vi "TemperatureProfileDesigner.vi"() -> (3 "ShcemeCluster":cluster{"Time":dbl, "Voltage":dbl}[](array[cluster]))   [LabVIEW 2023]
uses:
  <vilib>/Analysis/1siggen.llb/Ramp Pattern by Samples.vi
  <vilib>/Analysis/1siggen.llb/Ramp Pattern by Delta.vi
  <vilib>/Analysis/NI_AALBase.lvlib
panel:
  in  "Time (s)":dbl
  out "XY Graph":cluster{dbl[], dbl[]}(graph)
  in  "Schedule":bool
  in  "Ramp points (s)":i16 min=0 max=7200 step=1
  in  "Step / Ramp":bool
  in  "Up & Down":bool
  in  "Step":dbl min=0.0 max=450.0 step=1.0
  in  "Stop":dbl=20.0 min=20.0 max=450.0 step=1.0
  in  "Start":dbl=20.0 min=20.0 max=450.0 step=1.0
  # "Temperature Profile Designer"
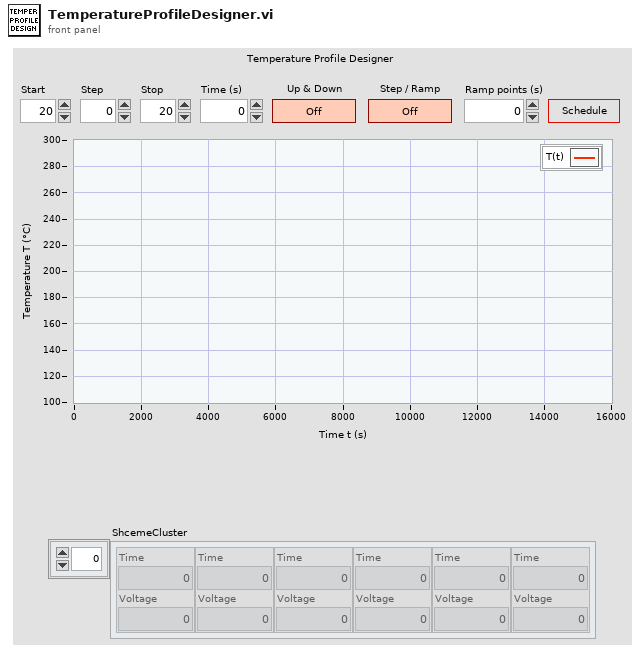
[diagram p1: front panel]
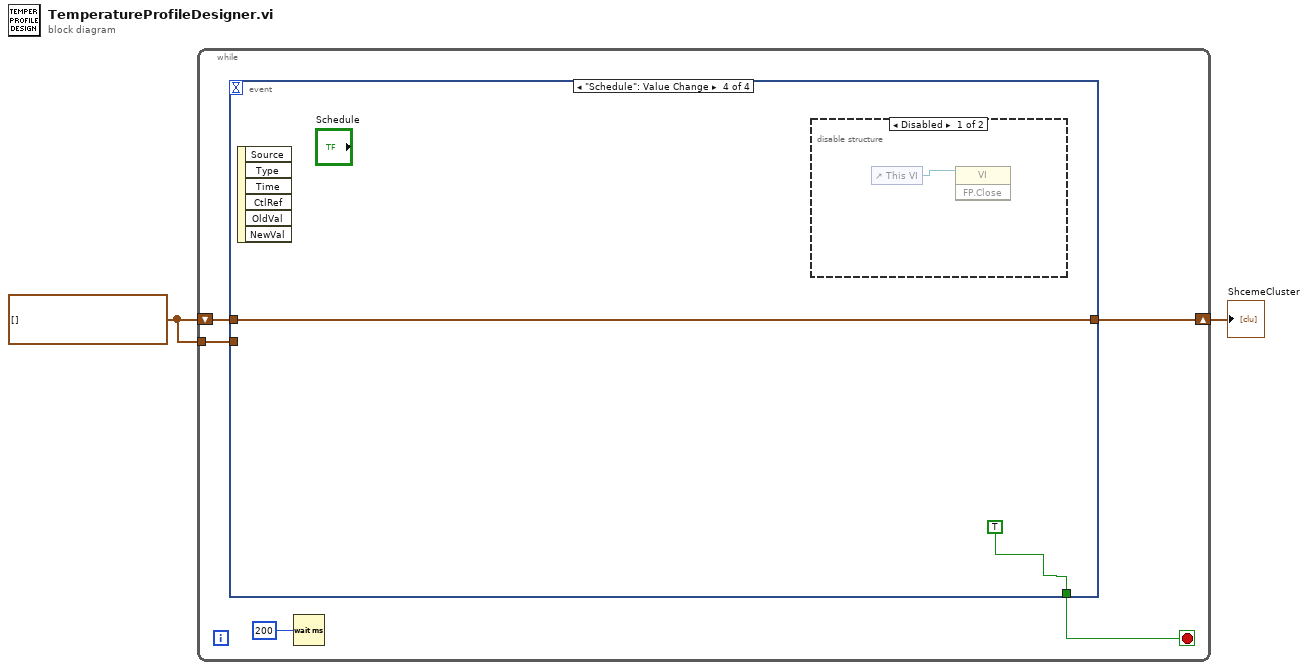
[diagram p0: block diagram]
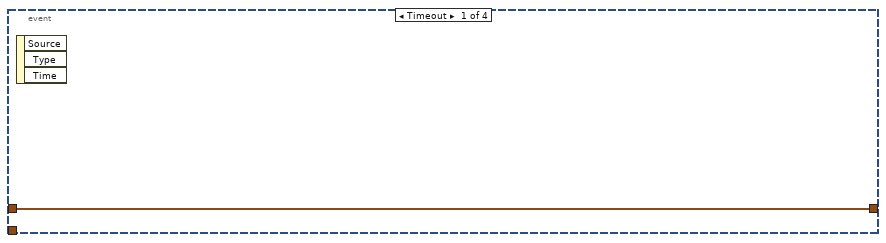
[diagram p2: hidden frame]
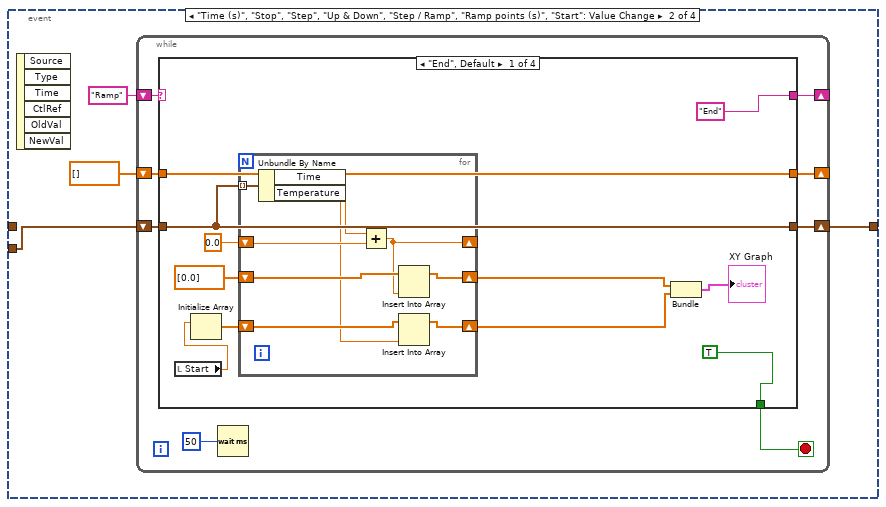
[diagram p3: hidden frame]
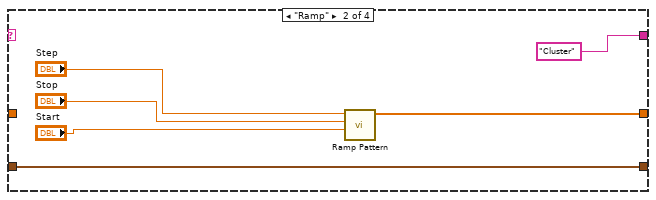
[diagram p4: hidden frame]
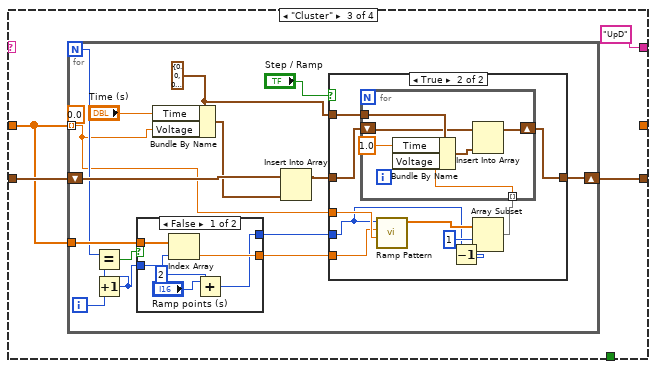
[diagram p5: hidden frame]
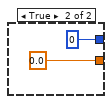
[diagram p6: hidden frame]
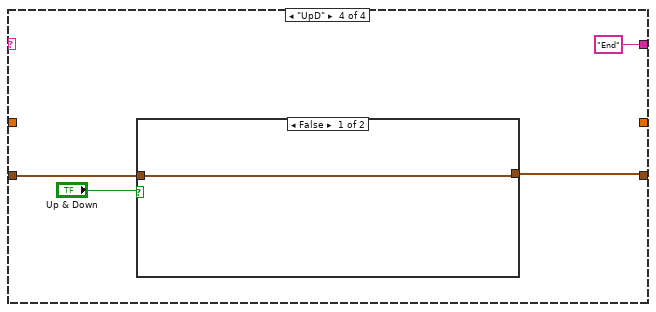
[diagram p8: hidden frame]
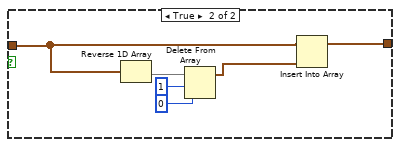
[diagram p9: hidden frame]
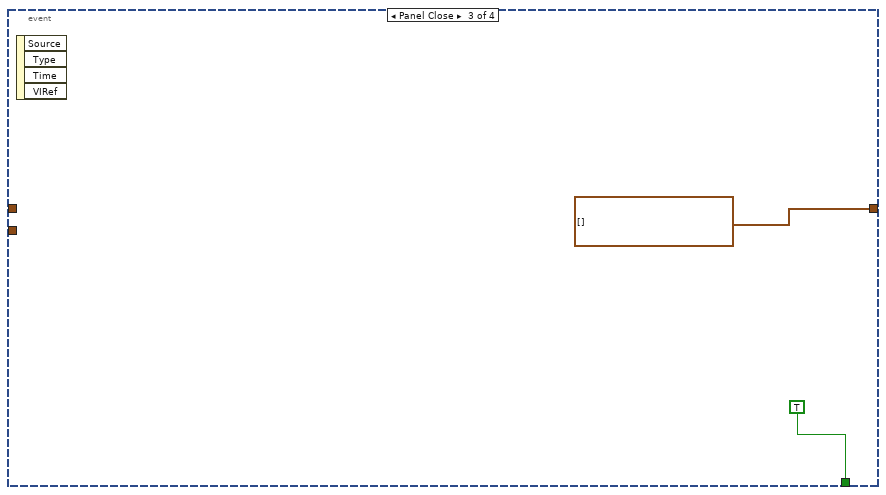
[diagram p10: hidden frame]
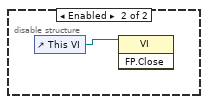
[diagram p11: hidden frame]
diagram:
  w1 = cluster{"Time":dbl, "Temperature":dbl}[] []
  n1 = while {
    shift-right: [w3] -> w2
    shift-left: w1 -> [w5]
    tunnel: w1 -> [w4]
    stop <- w6 stop-if-true
    n2 = event shown="[3] \"Schedule\": Value Change" {
      selector: _ -> [_ _ _ _]
      dyn-events: _ -> [_ _ _ _]
      timeout: _ -> [_ _ _ _]
      tunnel: [_ _ TRUE TRUE] -> w6
      tunnel: [w8 w10 cluster{"Time":dbl, "Temperature":dbl}[] [] w104] -> w3
      tunnel: w5 -> [w8 _ _ w104]
      tunnel: w4 -> [_ w9 _ _]
      event Timeout {
        n3 = event-data() -> ()  [unwired: 1 in, 3 out]
      }
      event "Time (s)", "Stop", "Step", "Up & Down", "Step / Ramp", "Ramp points (s)", "Start": Value Change {
        n4 = event-data() -> ()  [unwired: 1 in, 6 out]
        n5 = while {
          shift-right: [w19] -> _
          shift-left: "Ramp" -> [w20]
          shift-right: [w16] -> _
          shift-left: dbl[] [] ("Ramp Pattern") -> [w15]
          shift-right: [w13] -> w10
          shift-left: w9 -> [w14]
          stop <- w18 stop-if-true
          n6 = case shown="\"End\", Default" w20 {
            tunnel: ["End" "Cluster" "UpD" "End"] -> w19
            tunnel: [TRUE _ _ _] -> w18
            tunnel: [w29 w42 _ _] -> w16
            tunnel: w15 -> [w29 _ w48 _]
            tunnel: w14 -> [w28 w41 w50 w94]
            tunnel: [w28 w41 w49 w93] -> w13
            frame "End", Default {
              n7 = local read "Start"() -> (w26:dbl)
              n8 = Initialize Array(w26) -> (w25:dbl[])  [unwired: 1 in]
              n9 = for {
                tunnel: w28 -> [w40] mode=indexing
                shift-right: [w36] -> _
                shift-left: 0.0 -> [w38]
                shift-right: [w35] -> w23
                shift-left: dbl[] [0.0] ("Ramp Pattern") -> [w39]
                shift-right: [w34] -> w22
                shift-left: w25 -> [w33]
                n10 = Unbundle By Name(w40) -> ("Time"=w37:dbl, "Temperature"=w32:dbl)
                n11 = Add(x=w37, y=w38) -> (x+y=w36:dbl)
                n12 = Insert Into Array(array=w39, new element=w36) -> (w35:dbl[])  [unwired: 1 in]
                n13 = Insert Into Array(array=w33, new element=w32) -> (w34:dbl[])  [unwired: 1 in]
              }
              n14 = Bundle("Ramp Pattern"=w23, w22) -> (→"XY Graph":cluster{"Ramp Pattern":dbl[], dbl[]})  [unwired: 1 in]
            }
            frame "Ramp" {
              n15 = call-poly <vilib>:"Ramp Pattern.vi"("start"="Start", "end"="Stop", "delta"="Step") -> ("Ramp Pattern"=w42:dbl[])  [unwired: 6 in, 2 out]
            }
            frame "Cluster" {
              n16 = for {
                N -> [w57]
                tunnel: w48 -> [w53] mode=indexing
                shift-right: [w62] -> w49
                shift-left: w50 -> [w65]
                tunnel: w48 -> [w60]
                i -> [w52]
                (unwired) 0.0 ("f")
                w55 = cluster{"Time":dbl, "Voltage":dbl} {"Time"=0.0, "Voltage"=0.0}
                n17 = Increment(x=w52) -> (x+1=w58:i32)
                n18 = Equal?(x=w57, y=w58) -> (x = y?=w59:bool)
                n19 = case shown="False" w59 {
                  tunnel: w60 -> [w71 _]
                  tunnel: w58 -> [w70 _]
                  tunnel: [w69 0.0] -> w56
                  tunnel: [w66 i16 0 ("Ramp points (s)")] -> w54
                  frame False {
                    n20 = Index Array(array=w71, index=w70) -> (element=w69:dbl)
                    n21 = Add(x="Ramp points (s)", y=i16 2) -> (x+y=w66:i16)
                  }
                  frame True {
                  }
                }
                n22 = Bundle By Name(cluster=w55, "Time"="Time (s)", "Voltage"=w53) -> (w64:cluster{"Time":dbl, "Voltage":dbl})
                n23 = Insert Into Array(array=w65, new element=w64) -> (w61:cluster{"Time":dbl, "Temperature":dbl}[])  [unwired: 1 in]
                n24 = case shown="True" "Step / Ramp" {
                  tunnel: [w74 w81] -> w62
                  tunnel: w61 -> [w74 w82]
                  tunnel: w56 -> [_ w83]
                  tunnel: w53 -> [_ w84]
                  tunnel: w55 -> [_ w80]
                  tunnel: w54 -> [_ w76]
                  frame False {
                  }
                  frame True {
                    n25 = call-poly <vilib>:"Ramp Pattern.vi"("start"=w84, "end"=w83, "samples"=w76) -> ("Ramp Pattern"=w79:dbl[])  [unwired: 7 in, 1 out]
                    n26 = Decrement(x=w76) -> (x-1=w75:i16)
                    n27 = Array Subset(array=w79, index=1, length=w75) -> (w77:dbl[])
                    n28 = for {
                      shift-right: [w86] -> w81
                      shift-left: w82 -> [w88]
                      tunnel: w77 -> [w85] mode=indexing
                      tunnel: w80 -> [w89]
                      n29 = Bundle By Name(cluster=w89, "Time"=1.0, "Voltage"=w85) -> (w87:cluster{"Time":dbl, "Voltage":dbl})
                      n30 = Insert Into Array(array=w88, new element=w87) -> (w86:cluster{"Time":dbl, "Temperature":dbl}[])  [unwired: 1 in]
                    }
                  }
                }
              }
            }
            frame "UpD" {
              n31 = case shown="False" "Up & Down" {
                tunnel: w94 -> [w95 w98]
                tunnel: [w95 w96] -> w93
                frame False {
                }
                frame True {
                  n32 = Reverse 1D Array(array=w98) -> (reversed array=w101:cluster{"Time":dbl, "Temperature":dbl}[])
                  n33 = Delete From Array(array=w101, length=1, index=0) -> (array with subset deleted=w97:cluster{"Time":dbl, "Temperature":dbl}[])  [unwired: 1 out]
                  n34 = Insert Into Array(array=w98, new element=w97) -> (w96:cluster{"Time":dbl, "Temperature":dbl}[])  [unwired: 1 in]
                }
              }
            }
          }
          n35 = Wait (ms)(milliseconds to wait=u32 50) -> ()  [unwired: 1 out]
        }
      }
      event Panel Close {
        n36 = event-data() -> ()  [unwired: 1 in, 4 out]
      }
      event "Schedule": Value Change {
        n37 = event-data() -> ()  [unwired: 1 in, 6 out]
        n38 = disable-structure shown="Disabled" {
          frame Disabled {
            n39 = control-ref of="This VI"() -> (w106:refnum<vi>)
            n40 = invoke class="VI" method="FP.Close"(reference=w106) -> ()  [unwired: 2 in, 3 out]
          }
          frame Enabled {
            n41 = control-ref of="This VI"() -> (w107:refnum<vi>)
            n42 = invoke class="VI" method="FP.Close"(reference=w107) -> ()  [unwired: 2 in, 3 out]
          }
        }
      }
    }
    n43 = Wait (ms)(milliseconds to wait=u32 200) -> ()  [unwired: 1 out]
  }
  "ShcemeCluster" <- w2
